vi "VCM_ControlMonitor.vi"() -> ()   [LabVIEW 2018]
uses:
  Utility/Monitor Communication/Mischer/VCM-Cluster.ctl
  Global/Global Variables/Data_Display_global.vi
  Instrument_Setup.vi
panel:
  in  "Stopp":bool
  out "VCM Monitor":T1
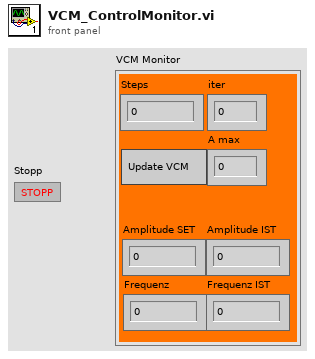
[diagram p1: front panel]
types:
  T1 = typedef "VCM-Cluster.ctl" = cluster{"Steps":dbl, "Amplitude SET":dbl, "Frequenz":dbl, "Amplitude IST":dbl, "Frequenz IST":dbl, "A max":dbl, "iter":dbl, "Update VCM":bool}
  T2 = cluster{"PE7265 AutoSens at ech step":bool, "PE7265 Sens":i32, "Coupling":bool, "AC Gain":u16, "Auto AC Gain":bool, "Input Device (Voltage Mode)":bool, "Line Frequency":bool, "Input Connector Shells":bool, "PE7265 Input Mode":u16, "Line Frequency\nRejection Filter":u8, "Port":u16, "7265 GPIB Address":i8, "Interface":bool, "Exit":bool, "GPIB Parameter 7260":cluster{"address":string, "delay time":dbl, "mode":i32}, "PE7265 delay after AS":dbl, "VISA session PE7265":refnum<visa-resource-name>, "Slope":u8, "Synchronous TC":bool, "Time Constant":u16, "Reference I/P":u8, "Reference\nHarmonic":u16, "Oscillator Amplitude (Volts rms)":dbl, "Oscillator Frequency (Hz)":dbl, "Ref Unlocked":bool, "Virtual Reference\nMode":bool}
  T3 = cluster{"address":string, "delay time":dbl, "mode":i32}
  T4 = typedef "VCM-Control.ctl" = cluster{"Steps":dbl, "Amplitude SET":dbl, "Frequenz":dbl, "A max":dbl, "Update VCM":bool}
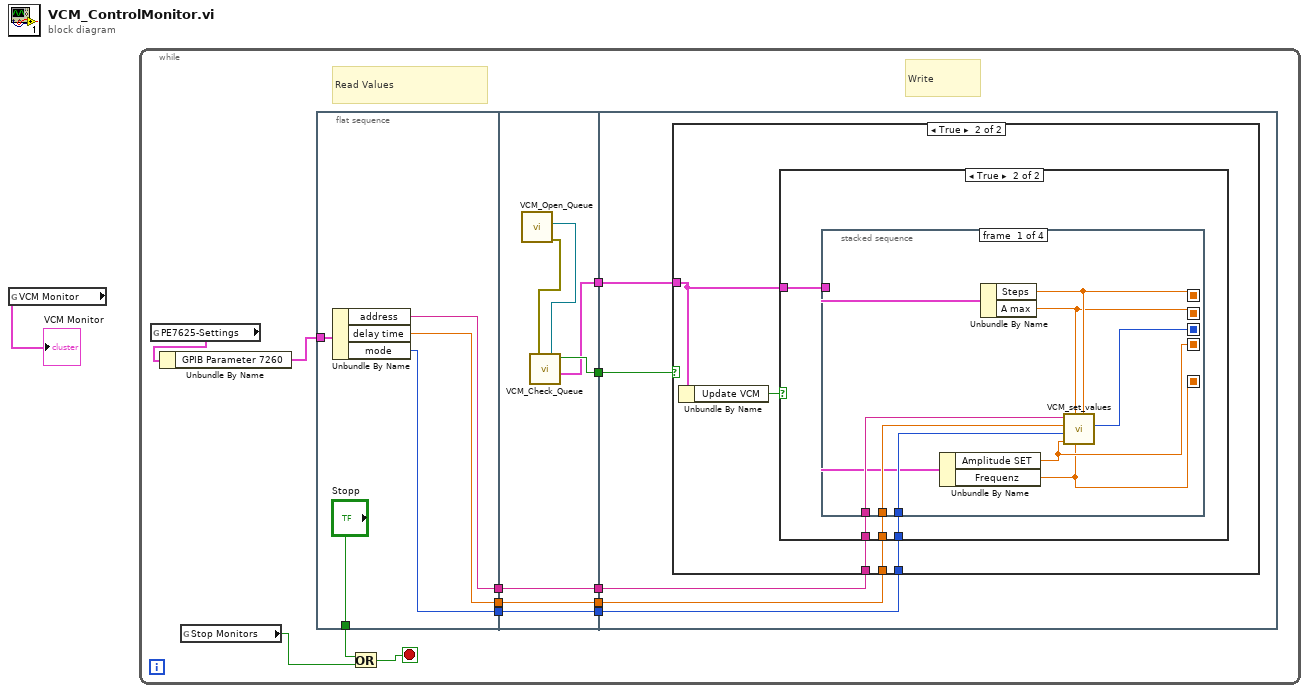
[diagram p0: block diagram]
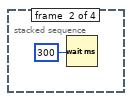
[diagram p4: hidden frame]
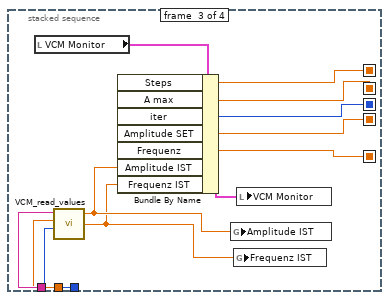
[diagram p5: hidden frame]
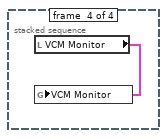
[diagram p6: hidden frame]
diagram:
  n1 = global read "Data_Display_global.vi" "VCM Monitor"() -> (→"VCM Monitor":T1)
  n2 = while {
    stop <- w4 stop-if-true
    # "Write"
    # "Read Values"
    n3 = global read "Instrument_Setup.vi" "PE7625-Settings"() -> (w8:T2)
    n4 = Unbundle By Name(w8) -> ("GPIB Parameter 7260"=w7:T3)
    n5 = global read "Data_Display_global.vi" "Stop Monitors"() -> (w5:bool)
    n6 = flat-sequence {
      tunnel: w7 -> [w19]
      tunnel: [w18] -> w13
      tunnel: [w17] -> w11
      tunnel: ["Stopp"] -> w6
      tunnel: [w15] -> w3
      tunnel: [w26] -> w14
      tunnel: w13 -> [w26]
      tunnel: [w25] -> w12
      tunnel: w11 -> [w25]
      tunnel: [w22] -> w10
      tunnel: [w21] -> w9
      tunnel: w3 -> [w20]
      tunnel: [w20] -> w2
      tunnel: w14 -> [w29]
      tunnel: w12 -> [w28]
      tunnel: w10 -> [w31]
      tunnel: w9 -> [w30]
      tunnel: w2 -> [w27]
      frame #0 {
        n7 = Unbundle By Name(w19) -> ("address"=w18:string, "delay time"=w17:dbl, "mode"=w15:i32)
      }
      frame #1 {
        n8 = call "VCM_Open_Queue.vi"() -> ("error out"=w24:errorcluster, "queue out"=w23:refnum<queue>)  [unwired: 10 in]
        n9 = call "VCM_Check_Queue.vi"("Error In"=w24, "queue"=w23) -> ("VCM Control"=w21:T4, "New Entries?"=w22:bool)  [unwired: 6 in, 1 out]
      }
      frame #2 {
        n10 = case shown="True" w31 {
          tunnel: w30 -> [_ w35]
          tunnel: w29 -> [_ w34]
          tunnel: w28 -> [_ w33]
          tunnel: w27 -> [_ w32]
          frame False {
          }
          frame True {
            n11 = Unbundle By Name(w35) -> ("Update VCM"=w36:bool)
            n12 = case shown="True" w36 {
              tunnel: w35 -> [_ w40]
              tunnel: w34 -> [_ w39]
              tunnel: w33 -> [_ w38]
              tunnel: w32 -> [_ w37]
              frame False {
              }
              frame True {
                n13 = stacked-sequence {
                  seq-local: [w49 _ _ _] -> [_ _ w55 _]
                  seq-local: [w48 _ _ _] -> [_ _ w57 _]
                  seq-local: [w47 _ _ _] -> [_ _ w56 _]
                  seq-local: [w42 _ _ _] -> [_ _ w54 _]
                  seq-local: [w41 _ _ _] -> [_ _ w53 _]
                  tunnel: w40 -> [w43 _ _ _]
                  tunnel: w39 -> [w46 _ w62 _]
                  tunnel: w38 -> [w45 _ w61 _]
                  tunnel: w37 -> [w44 _ w60 _]
                  frame #0 {
                    n14 = Unbundle By Name(w43) -> ("Amplitude SET"=w42:dbl, "Frequenz"=w41:dbl)
                    n15 = Unbundle By Name(w43) -> ("Steps"=w48:dbl, "A max"=w47:dbl)
                    n16 = call "VCM_set_values.vi"("Steps"=w48, "Frequenz"=w41, "A max"=w47, "Amplitude SET"=w42, "mode"=w44, "delay time"=w45, "address"=w46) -> ("iter"=w49:i32)  [unwired: 2 in, 1 out]
                  }
                  frame #1 {
                    n17 = Wait (ms)(milliseconds to wait=300) -> ()  [unwired: 1 out]
                  }
                  frame #2 {
                    n18 = local read "VCM Monitor"() -> (w59:T1)
                    n19 = call "VCM_read_values.vi"("mode"=w60, "delay time"=w61, "address"=w62) -> ("Frequenz IST"=w51:dbl, "Amplitude IST"=w52:dbl)  [unwired: 2 in]
                    n20 = Bundle By Name(cluster=w59, "Steps"=w57, "A max"=w56, "iter"=w55, "Amplitude SET"=w54, "Frequenz"=w53, "Amplitude IST"=w52, "Frequenz IST"=w51) -> (w58:T1)
                    n21 = global write "Instrument_Setup.vi" "Amplitude IST"(w52) -> ()
                    n22 = global write "Instrument_Setup.vi" "Frequenz IST"(w51) -> ()
                    n23 = local write "VCM Monitor"(w58) -> ()
                  }
                  frame #3 {
                    n24 = local read "VCM Monitor"() -> (w63:T1)
                    n25 = global write "Data_Display_global.vi" "VCM Monitor"(w63) -> ()
                  }
                }
              }
            }
          }
        }
      }
    }
    n26 = Or(x=w6, y=w5) -> (x .or. y?=w4:bool)
  }
